vi "Write MusicLibrary.vi"(8 "error in (no error)":errorcluster, 10 "MusicLibrary.lvclass":refnum<class "MusicLibrary.lvclass">, 11 "MusicFile in":refnum<class "MusicFile.lvclass">) -> (0 "error out":errorcluster, 3 "MusicFile out":refnum<class "MusicFile.lvclass">)   [LabVIEW 2015, in "MusicFile.lvclass"]
uses:
  MusicFile.lvclass
  MusicElementLibrary/MusicLibrary/MusicLibrary.lvclass
  MusicFile.lvclass/MusicFile.ctl
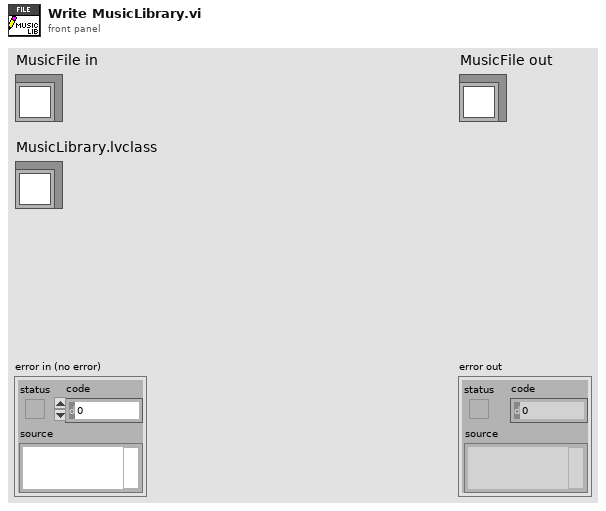
[diagram p1: front panel]
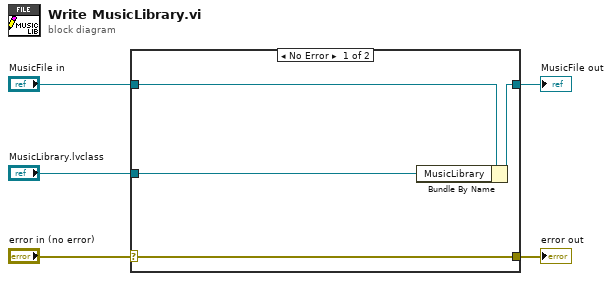
[diagram p0: block diagram]
diagram:
  n1 = case shown="No Error" "error in (no error)" {
    selector: "error in (no error)" -> [w9 w10]
    tunnel: [w9 w10] -> w4
    tunnel: [w7 w11] -> w2
    tunnel: "MusicFile in" -> [w8 w11]
    tunnel: "MusicLibrary.lvclass" -> [w6 _]
    frame No Error {
      n2 = Bundle By Name(cluster=w8, "MusicLibrary"=w6) -> (w7:refnum<class "MusicFile.lvclass">)
    }
    frame Error {
    }
  }
  "error out" <- w4
  "MusicFile out" <- w2
